vi "Set Subject and Body of MailMessage.vi"(8 "error in (no error)":errorcluster caption="错误输入（无错误）", 9 "Body":string, 10 "Subject":string, 11 "Email In":refnum<class "Email.lvclass"> caption="DNL_LabVIEW Object in") -> (0 "error out":errorcluster caption="错误输出", 3 "Email Out":refnum<class "Email.lvclass"> caption="DNL_LabVIEW Object out")   [LabVIEW 2012, in "Email.lvclass"]
uses:
  Email.lvclass
  Email.lvclass/Email.ctl
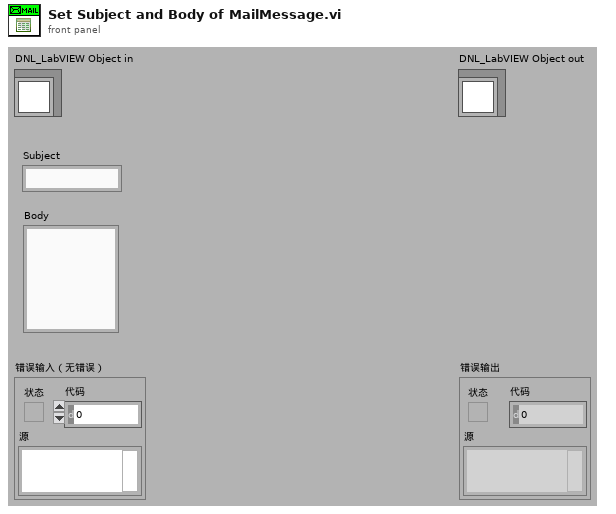
[diagram p1: front panel]
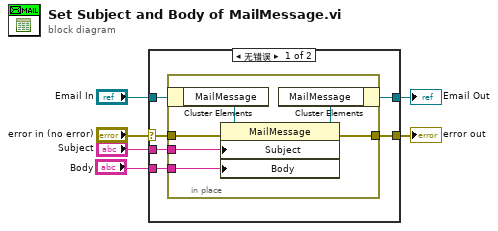
[diagram p0: block diagram]
diagram:
  n1 = case shown="无错误" "error in (no error)" {
    selector: "error in (no error)" -> [w11 w20]
    tunnel: [w10 w20] -> w5
    tunnel: [w7 w19] -> w3
    tunnel: "Email In" -> [w12 w19]
    tunnel: "Subject" -> [w9 _]
    tunnel: "Body" -> [w8 _]
    frame No Error {
      n2 = in-place {
        in-place-border: w11 -> [w16]
        in-place-border: [w15] -> w10
        in-place-border: w9 -> [w14]
        in-place-border: w8 -> [w13]
        n3 = in-place-cluster #1(w12) -> ("MailMessage"=w18:refnum<k24>)
        n4 = property class="MailMessage"(reference=w18, error in=w16, "Subject"=w14, "Body"=w13) -> (reference out=w17:refnum<k24>, error out=w15:errorcluster)
        n5 = in-place-cluster #1("MailMessage"=w17) -> (w7:refnum<class "Email.lvclass">)
      }
    }
    frame Error {
    }
  }
  "error out" <- w5
  "Email Out" <- w3
